vi "Maya2000 - Open all.vi"(8 "error in (no error)":errorcluster, 10 "Maya reference in":refnum<k24>, 11 "Maya2000 Basic\n[UV2400,UV600] in":T1[](array[typedef])) -> (0 "error out":errorcluster, 2 ".NET Refnum out":refnum<k24>, 3 "Maya2000 Basic \n[UV2400,UV600]":T1[](array[typedef]))   [LabVIEW 2016]
uses:
  Maya2000 Typedefs/Maya2000 basic info.ctl
  C:/Program Files/Ocean Optics/OmniDriver/OOI_HOME/NETOmniDriver-NET40.dll
  Program Files/Ocean Optics/OmniDriver/OOI_HOME/NETOmniDriver-NET40.dll
panel:
  in  "Maya basic":T1
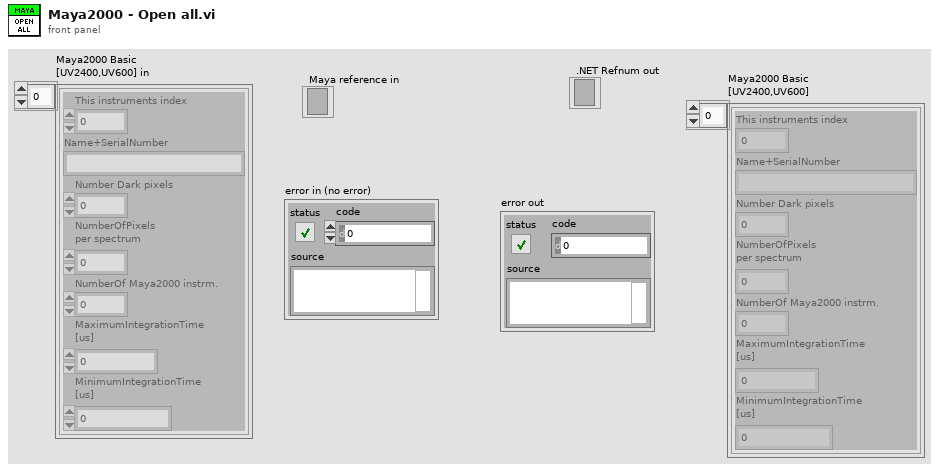
[diagram p1: front panel]
types:
  T1 = typedef "Maya2000 basic info.ctl" = cluster{"This instruments index":i32, "Name+SerialNumber":string, "Number Dark pixels":i32, "NumberOfPixels\nper spectrum":i32, "NumberOf Maya2000 instrm.":i32, "MaximumIntegrationTime\n[us]":i32, "MinimumIntegrationTime\n[us]":i32}
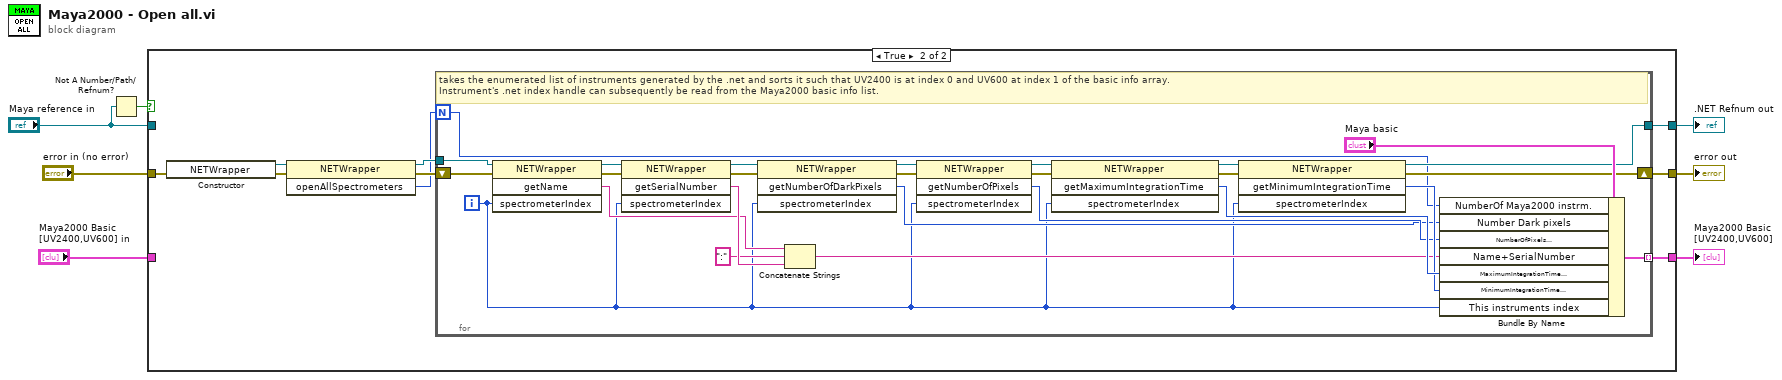
[diagram p0: block diagram]
diagram:
  n1 = Not A Number/Path/Refnum?(number/path/refnum="Maya reference in") -> (NaN/Path/Refnum?=w2:bool)
  n2 = case shown="True" w2 {
    tunnel: "error in (no error)" -> [w8 w15]
    tunnel: [w9 w13] -> w6
    tunnel: [w10 w12] -> w5
    tunnel: "Maya2000 Basic\n[UV2400,UV600] in" -> [w10 _]
    tunnel: "Maya reference in" -> [w9 _]
    tunnel: [w8 w11] -> w1
    frame False {
    }
    frame True {
      n3 = constructor class="NETWrapper"(error in=w15) -> (reference out=w17:refnum<k24>, error out=w16:errorcluster)  [unwired: 2 in, 1 out]
      n4 = invoke class="NETWrapper" method="openAllSpectrometers"(reference=w17, error in=w16) -> (reference out=w19:refnum<k24>, error out=w18:errorcluster, "openAllSpectrometers"=w14:i32)  [unwired: 1 in]
      n5 = for {
        N: w14 -> [w21]
        tunnel: w19 -> [w45]
        tunnel: [w26] -> w13
        shift-right: [w25] -> w11
        shift-left: w18 -> [w44]
        tunnel: [w20] -> w12 mode=indexing
        i -> [w22]
        # "takes the enumerated list of instruments generated by the .net and sorts it such that UV2400 is at index 0 and UV600 at index 1 of the basic info array.\nInstrument's .net index handle can subsequently be read from the Maya2000 basic info list."
        n6 = invoke class="NETWrapper" method="getName"(reference=w45, error in=w44, "spectrometerIndex"=w22) -> (reference out=w28:refnum<k24>, error out=w27:errorcluster, "getName"=w29:string)  [unwired: 1 in, 1 out]
        n7 = invoke class="NETWrapper" method="getSerialNumber"(reference=w28, error in=w27, "spectrometerIndex"=w22) -> (reference out=w33:refnum<k24>, error out=w32:errorcluster, "getSerialNumber"=w31:string)  [unwired: 1 in, 1 out]
        n8 = invoke class="NETWrapper" method="getNumberOfDarkPixels"(reference=w33, error in=w32, "spectrometerIndex"=w22) -> (reference out=w34:refnum<k24>, error out=w35:errorcluster, "getNumberOfDarkPixels"=w40:i32)  [unwired: 1 in, 1 out]
        n9 = Concatenate Strings(w29, ":" ("string"), w31) -> (w38:string)
        n10 = invoke class="NETWrapper" method="getNumberOfPixels"(reference=w34, error in=w35, "spectrometerIndex"=w22) -> (reference out=w37:refnum<k24>, error out=w36:errorcluster, "getNumberOfPixels"=w41:i32)  [unwired: 1 in, 1 out]
        n11 = invoke class="NETWrapper" method="getMaximumIntegrationTime"(reference=w37, error in=w36, "spectrometerIndex"=w22) -> (reference out=w23:refnum<k24>, error out=w24:errorcluster, "getMaximumIntegrationTime"=w43:i32)  [unwired: 1 in, 1 out]
        n12 = invoke class="NETWrapper" method="getMinimumIntegrationTime"(reference=w23, error in=w24, "spectrometerIndex"=w22) -> (reference out=w26:refnum<k24>, error out=w25:errorcluster, "getMinimumIntegrationTime"=w42:i32)  [unwired: 1 in, 1 out]
        n13 = Bundle By Name(cluster="Maya basic", "NumberOf Maya2000 instrm."=w21, "Number Dark pixels"=w40, "NumberOfPixels\nper spectrum"=w41, "Name+SerialNumber"=w38, "MaximumIntegrationTime\n[us]"=w43, "MinimumIntegrationTime\n[us]"=w42, "This instruments index"=w22) -> (w20:T1)
      }
    }
  }
  ".NET Refnum out" <- w6
  "Maya2000 Basic \n[UV2400,UV600]" <- w5
  "error out" <- w1
